vi "SetMoveTolerance.vi"(1 "Traverse Name":string) -> (0 "Max Error in Eng Units":u32)   [LabVIEW 2018]
uses:
  Anemometry/Anemometry Sub Vis/Globals/Constants_global.vi
  <vilib>/Utility/config.llb/Read Key (U32).vi
  <vilib>/Utility/config.llb/Write Key (U32).vi
  <vilib>/Utility/config.llb/NI_LVConfig.lvlib
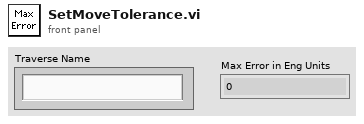
[diagram p1: front panel]
types:
  T1 = typedef "NI_LVConfig.lvlib/Config Data RefNum.ctl" = refnum<k1>
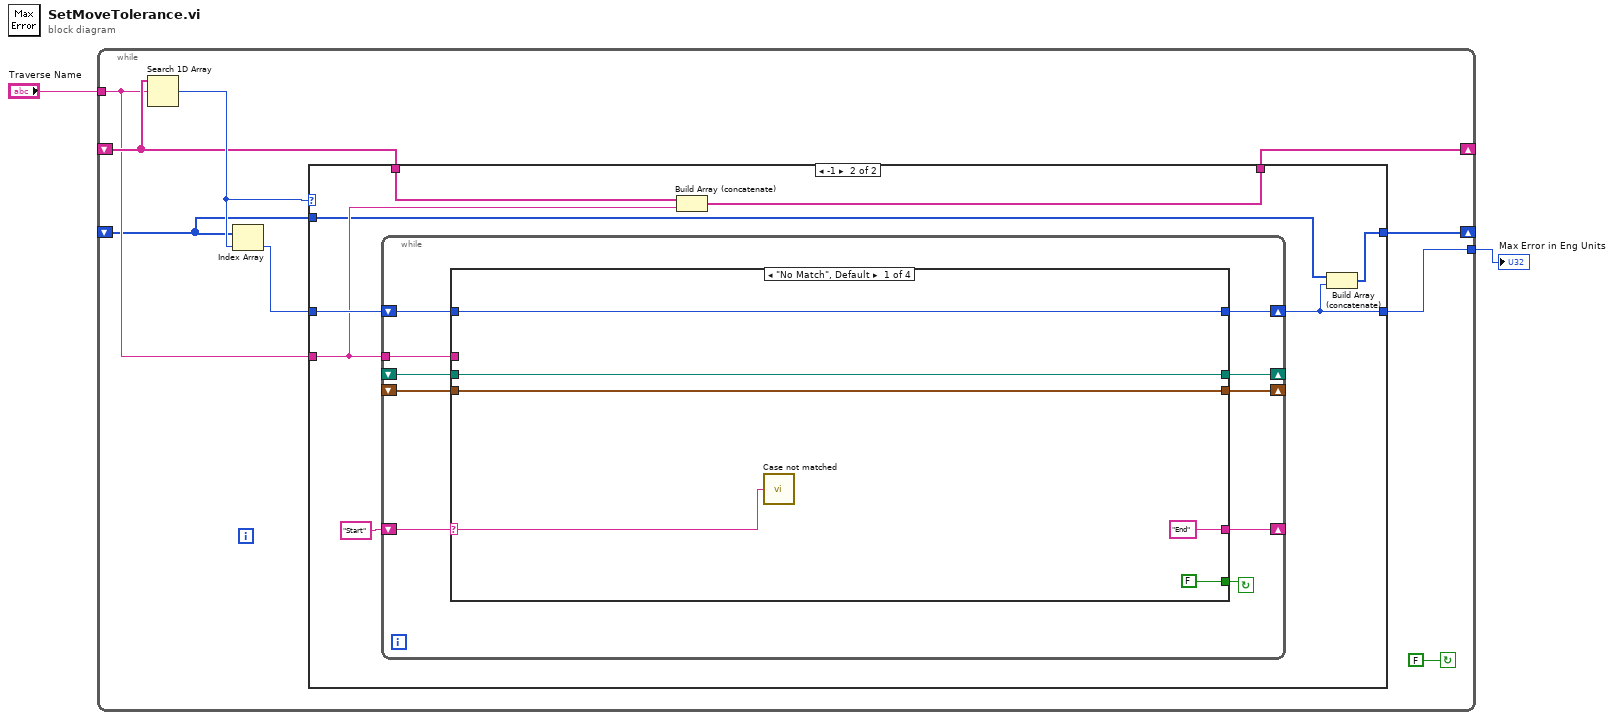
[diagram p0: block diagram]
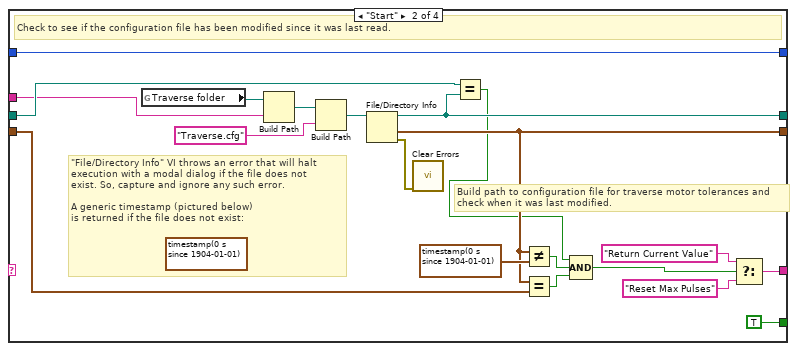
[diagram p3: hidden frame]
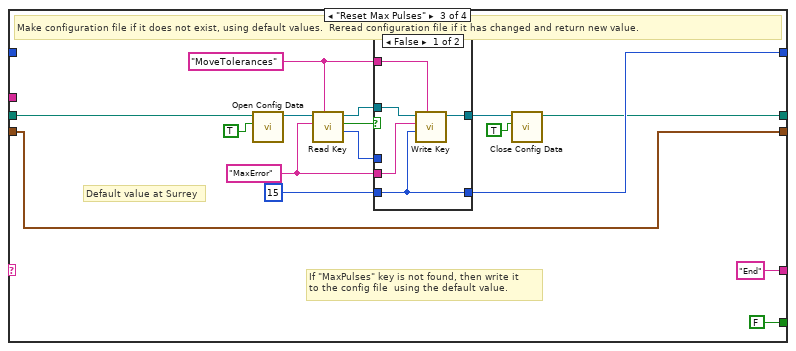
[diagram p4: hidden frame]
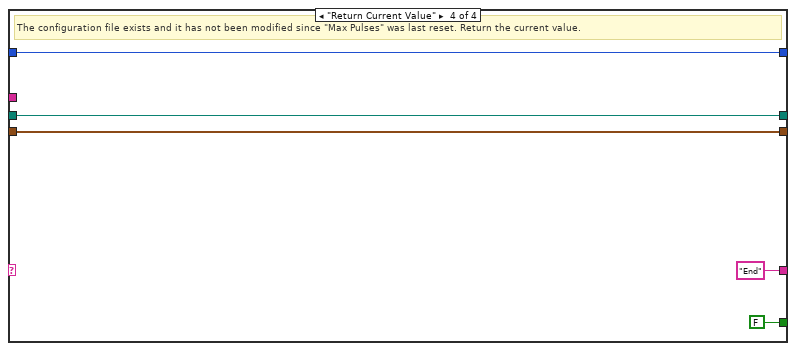
[diagram p6: hidden frame]
diagram:
  n1 = while {
    shift-right: [w6] -> _
    shift-left: _ -> [w7]
    tunnel: "Traverse Name" -> [w4]
    shift-right: [w9] -> _
    shift-left: _ -> [w3]
    tunnel: [w10] -> w1
    stop <- FALSE continue-if-true
    n2 = Search 1D Array(1D array=w7, element=w4) -> (index of element=w8:i32)  [unwired: 1 in]
    n3 = Index Array(array=w3, index=w8) -> (element=w11:u32)
    n4 = case shown="-1" w8 {
      tunnel: w4 -> [_ w19]
      tunnel: w11 -> [w14 w22]
      tunnel: [w14 w17] -> w10
      tunnel: [w12 w16] -> w9
      tunnel: w7 -> [w13 w20]
      tunnel: [w13 w18] -> w6
      tunnel: w3 -> [w12 w15]
      frame 0, Default {
      }
      frame -1 {
        n5 = while {
          tunnel: w19 -> [w29]
          shift-right: [w32] -> _
          shift-left: "Start" -> [w26]
          shift-right: [w24] -> _
          shift-left: _ -> [w30]
          shift-right: [w23] -> _
          shift-left: _ -> [w31]
          shift-right: [w27] -> w17
          shift-left: w22 -> [w28]
          stop <- w25 continue-if-true
          n6 = case shown="\"No Match\", Default" w26 {
            selector: w26 -> [w33 _ _ _]
            tunnel: [FALSE TRUE FALSE FALSE] -> w25
            tunnel: ["End" w50 "End" "End"] -> w32
            tunnel: [w36 w53 w63 w86] -> w27
            tunnel: [w35 w47 w60 w85] -> w23
            tunnel: w28 -> [w36 w53 _ w86]
            tunnel: w31 -> [w35 w49 w60 w85]
            tunnel: [w34 w42 w61 w82] -> w24
            tunnel: w30 -> [w34 w41 w62 w82]
            tunnel: w29 -> [_ w39 _ _]
            frame "No Match", Default {
              n7 = call "Case not matched.vi"("Case Name not Matched"=w33) -> ()
            }
            frame "Start" {
              (unwired) timestamp(0 s since 1904-01-01) ("last mod")
              # "Build path to configuration file for traverse motor tolerances and check when it was last modified."
              # "Check to see if the configuration file has been modified since it was last read."
              # "\"File/Directory Info\" VI throws an error that will halt execution with a modal dialog if the file does not \nexist. So, capture and ignore any such error.\n\nA generic timestamp (pictured below) is returned if the file does not exist:"
              # "\"File/Directory Info\" VI throws an error that will halt execution with a modal dialog if the file does not \nexist. So, capture and ignore any such error.\n\nA generic timestamp (pictured below)\nis returned if the file does not exist:"
              # "\"File/Directory Info\" VI throws an error that will halt execution with a modal dialog if the file does not \nexist. So, capture and ignore any such error.\n\nA generic timestamp (pictured below)\nis returned if the file does not exist:"
              n8 = global read "Constants_global.vi" "Traverse folder"() -> (w58:path)
              n9 = Build Path(base path=w58, name or relative path=w39) -> (appended path=w56:path)
              n10 = Build Path(base path=w56, name or relative path="Traverse.cfg") -> (appended path=w55:path)
              n11 = File/Directory Info(path=w55) -> (path out=w42:path, last mod=w47:timestamp, error out=w54:errorcluster)  [unwired: 1 in, 4 out]
              n12 = call <vilib>:"Clear Errors.vi"("error in (no error)"=w54) -> ()  [unwired: 5 in, 2 out]
              n13 = Equal?(x=w41, y=w42) -> (x = y?=w40:bool)
              n14 = Not Equal?(x=w47, y=timestamp(0 s since 1904-01-01) ("last mod")) -> (x != y?=w46:bool)
              n15 = Equal?(x=w47, y=w49) -> (x = y?=w45:bool)
              n16 = Compound Arithmetic op=AND(w40, w46, w45) -> (w51:bool)
              n17 = Select(t="Return Current Value", s=w51, f="Reset Max Pulses") -> (s? t:f=w50:string)
            }
            frame "Reset Max Pulses" {
              w70 = "MoveTolerances" ("section")
              w69 = "MaxError" ("key")
              # "If \"MaxPulses\" key is not found, then write it\nto the config file  using the default value."
              # "Default value at Surrey"
              # "Make configuration file if it does not exist, using default values.  Reread configuration file if it has changed and return new value."
              n18 = call <vilib>:"Open Config Data.vi"("create file if necessary (T)"=TRUE, "configuration file path"=w62) -> ("refnum"=w66:T1)  [unwired: 7 in, 2 out]
              n19 = call-poly <vilib>:"Read Key.vi"("section"=w70, "key"=w69, "refnum"=w66) -> ("value"=w68:u32, "found?"=w67:bool, "refnum out"=w72:T1)  [unwired: 5 in, 1 out]
              n20 = case shown="False" w67 {
                tunnel: w68 -> [_ w81]
                tunnel: w69 -> [w77 _]
                tunnel: w70 -> [w78 _]
                tunnel: u32 15 ("value") -> [w76 _]
                tunnel: [w76 w81] -> w63
                tunnel: w72 -> [w79 w80]
                tunnel: [w75 w80] -> w64
                frame False {
                  n21 = call-poly <vilib>:"Write Key.vi"("section"=w78, "value"=w76, "key"=w77, "refnum"=w79) -> ("refnum out"=w75:T1)  [unwired: 5 in, 2 out]
                }
                frame True {
                }
              }
              n22 = call <vilib>:"Close Config Data.vi"("write file if changed (T)"=TRUE, "refnum"=w64) -> ("file path"=w61:path)  [unwired: 8 in, 1 out]
            }
            frame "Return Current Value" {
              # "The configuration file exists and it has not been modified since \"Max Pulses\" was last reset. Return the current value."
            }
          }
        }
        n23 = Build Array (concatenate)(w20, w19) -> (w18:string[])
        n24 = Build Array (concatenate)(w15, w17) -> (w16:u32[])
      }
    }
  }
  "Max Error in Eng Units" <- w1
